vi "generate_RT_average.vi"(2 "Data In":T4, 7 "Variables Cluster":T2) -> (13 "Complete Data Out":T1, 15 "error out":errorcluster)   [LabVIEW 2023]
panel:
  out "C2 RT Avg Data":T3
  out "C1 RT Avg Data":T3
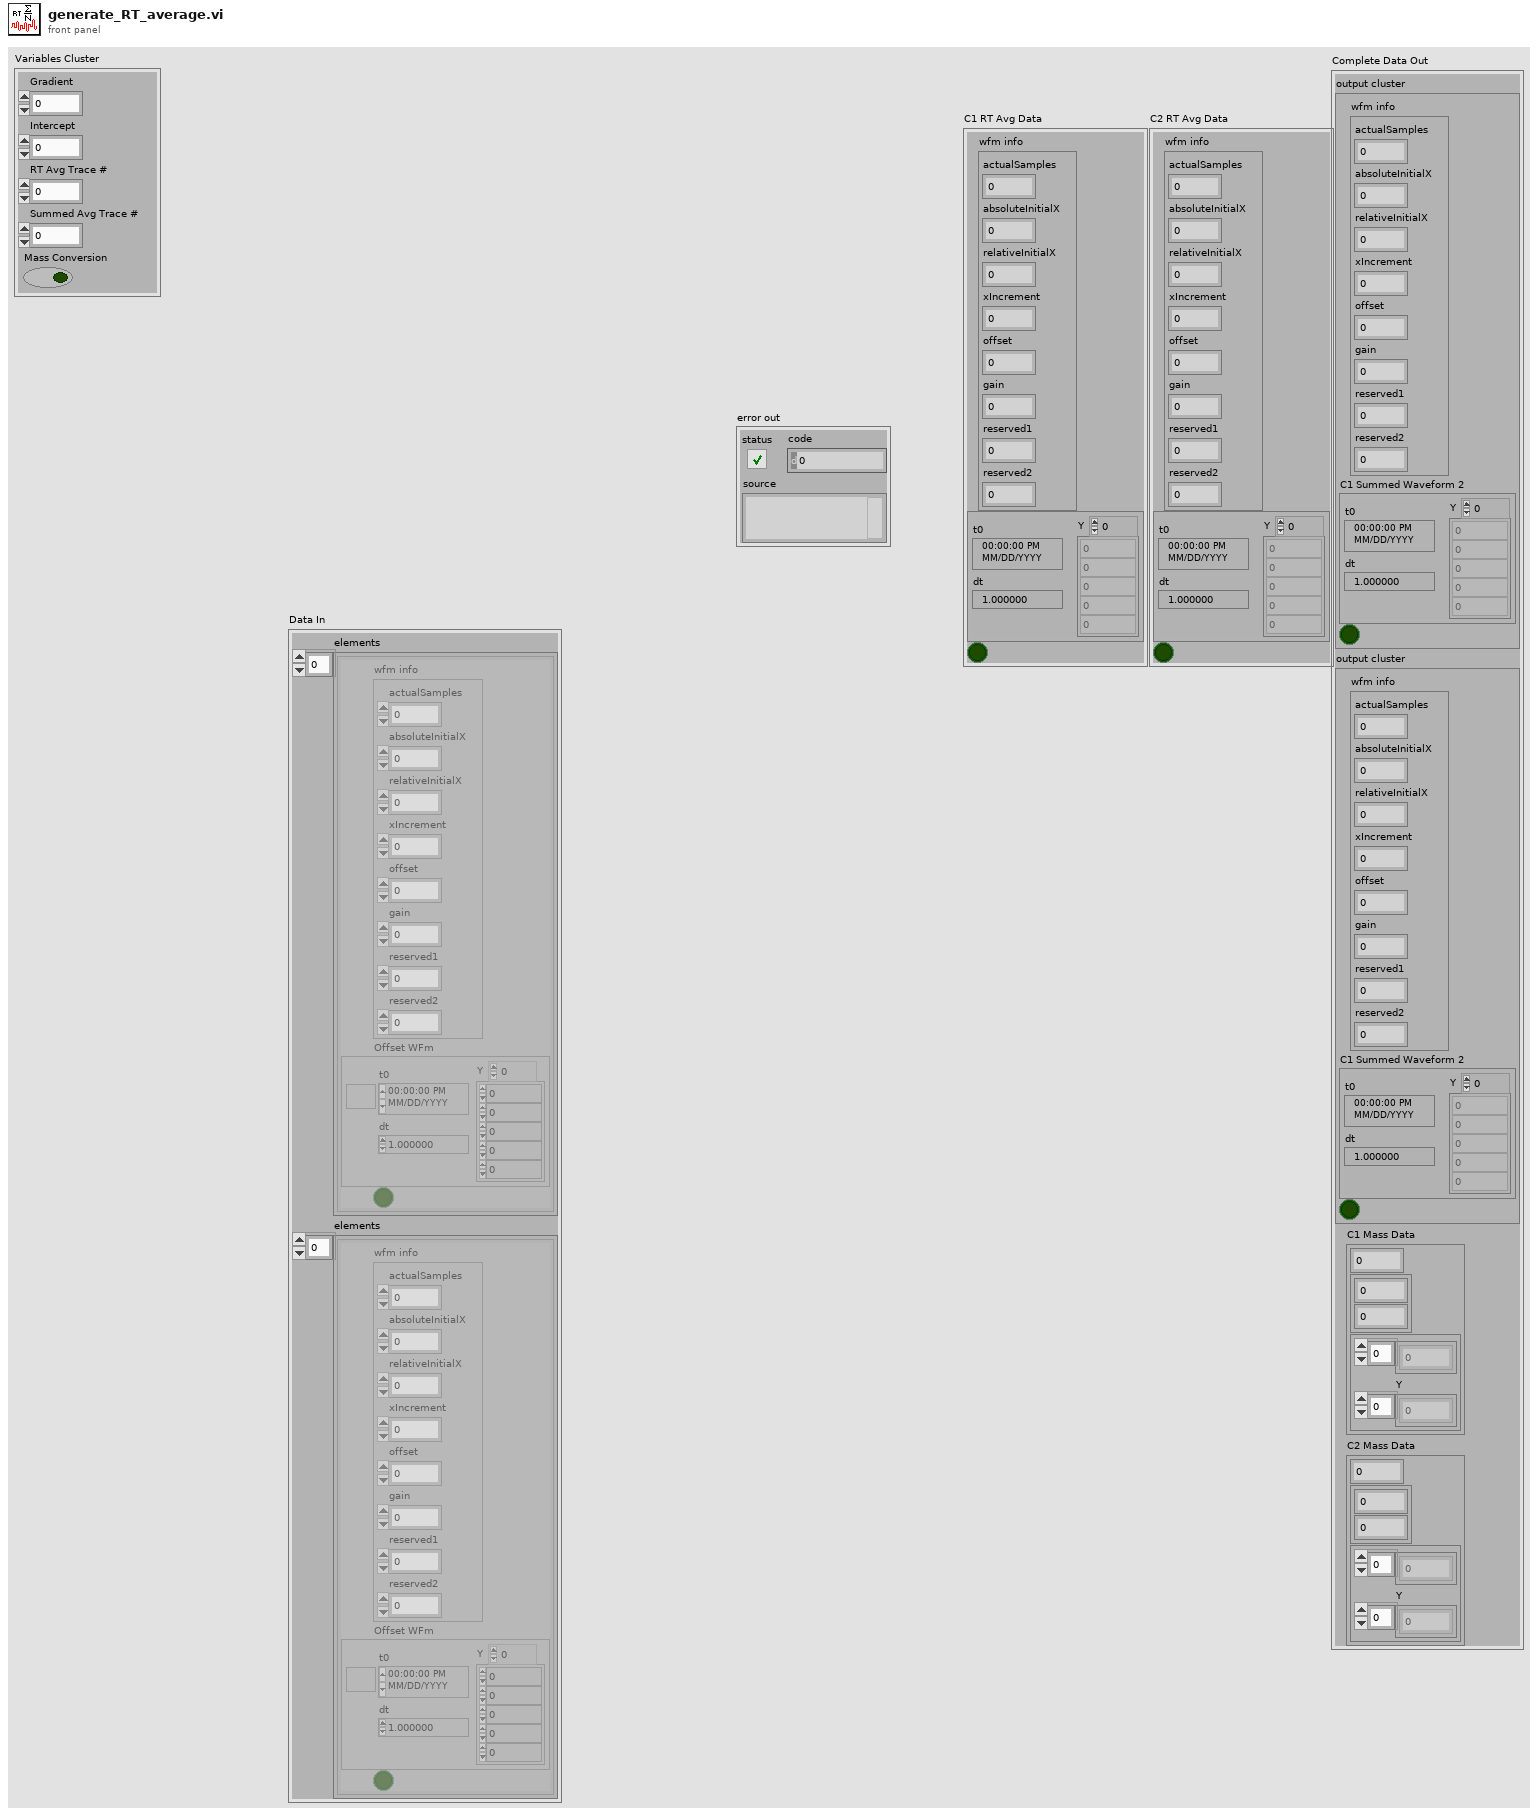
[diagram p1: front panel]
types:
  T1 = cluster{"output cluster":cluster{"wfm info":cluster{"actualSamples":i32, "absoluteInitialX":dbl, "relativeInitialX":dbl, "xIncrement":dbl, "offset":dbl, "gain":dbl, "reserved1":dbl, "reserved2":dbl}, "C1 Summed Waveform 2":waveform(dbl), bool}, "output cluster":cluster{"wfm info":cluster{"actualSamples":i32, "absoluteInitialX":dbl, "relativeInitialX":dbl, "xIncrement":dbl, "offset":dbl, "gain":dbl, "reserved1":dbl, "reserved2":dbl}, "C1 Summed Waveform 2":waveform(dbl), bool}, "C1 Mass Data":cluster{dbl, cluster{dbl, dbl}, cluster{dbl[], "Y":dbl[]}}, "C2 Mass Data":cluster{dbl, cluster{dbl, dbl}, cluster{dbl[], "Y":dbl[]}}}
  T2 = cluster{"Gradient":dbl, "Intercept":dbl, "RT Avg Trace #":i32, "Summed Avg Trace #":i32, "Mass Conversion":bool}
  T3 = cluster{"wfm info":cluster{"actualSamples":i32, "absoluteInitialX":dbl, "relativeInitialX":dbl, "xIncrement":dbl, "offset":dbl, "gain":dbl, "reserved1":dbl, "reserved2":dbl}, "Waveform":waveform(dbl), bool}
  T4 = cluster{"elements":cluster{"wfm info":cluster{"actualSamples":i32, "absoluteInitialX":dbl, "relativeInitialX":dbl, "xIncrement":dbl, "offset":dbl, "gain":dbl, "reserved1":dbl, "reserved2":dbl}, "Offset WFm":waveform(dbl), bool}[], "elements":cluster{"wfm info":cluster{"actualSamples":i32, "absoluteInitialX":dbl, "relativeInitialX":dbl, "xIncrement":dbl, "offset":dbl, "gain":dbl, "reserved1":dbl, "reserved2":dbl}, "Offset WFm":waveform(dbl), bool}[]}
  T5 = cluster{"wfm info":cluster{"actualSamples":i32, "absoluteInitialX":dbl, "relativeInitialX":dbl, "xIncrement":dbl, "offset":dbl, "gain":dbl, "reserved1":dbl, "reserved2":dbl}, "Offset WFm":waveform(dbl), bool}[]
  T6 = cluster{"actualSamples":i32, "absoluteInitialX":dbl, "relativeInitialX":dbl, "xIncrement":dbl, "offset":dbl, "gain":dbl, "reserved1":dbl, "reserved2":dbl}
  T7 = cluster{"wfm info":cluster{"actualSamples":i32, "absoluteInitialX":dbl, "relativeInitialX":dbl, "xIncrement":dbl, "offset":dbl, "gain":dbl, "reserved1":dbl, "reserved2":dbl}, waveform(dbl), bool}
  T8 = cluster{dbl, cluster{dbl, dbl}, cluster{dbl[], "Y":dbl[]}}
  T9 = cluster{cluster{"wfm info":cluster{"actualSamples":i32, "absoluteInitialX":dbl, "relativeInitialX":dbl, "xIncrement":dbl, "offset":dbl, "gain":dbl, "reserved1":dbl, "reserved2":dbl}, waveform(dbl), bool}, cluster{"wfm info":cluster{"actualSamples":i32, "absoluteInitialX":dbl, "relativeInitialX":dbl, "xIncrement":dbl, "offset":dbl, "gain":dbl, "reserved1":dbl, "reserved2":dbl}, waveform(dbl), bool}, "C1 Mass Data":cluster{dbl, cluster{dbl, dbl}, cluster{dbl[], "Y":dbl[]}}, "C2 Mass Data":cluster{dbl, cluster{dbl, dbl}, cluster{dbl[], "Y":dbl[]}}}
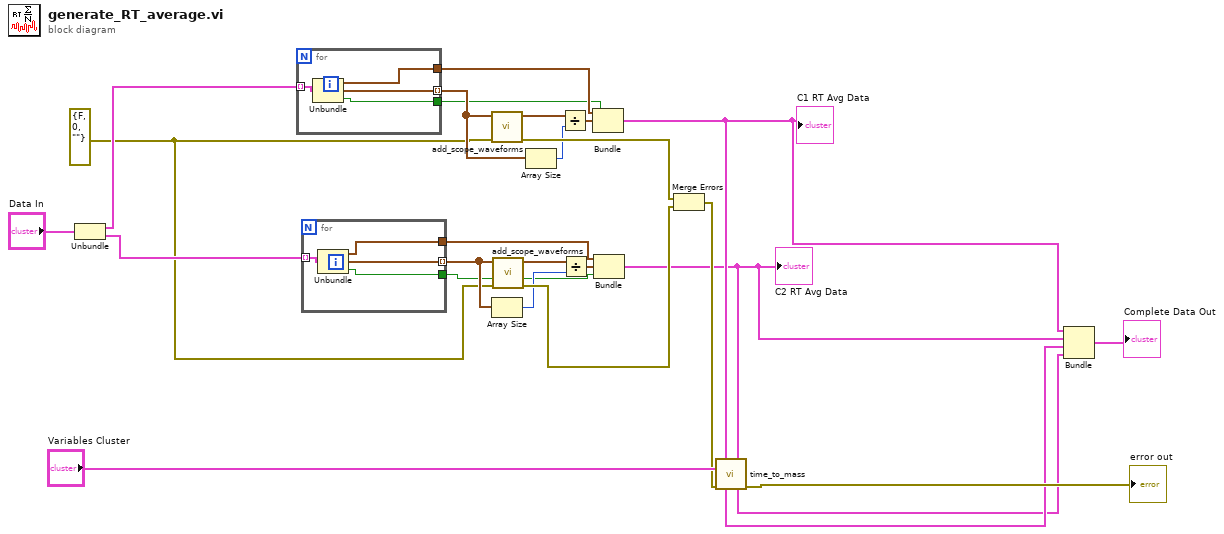
[diagram p0: block diagram]
diagram:
  w9 = errorcluster {"status"=FALSE, "code"=0, "source"=""} ("Error in (no error)")
  n1 = Unbundle("Data In") -> ("elements"=w26:T5, "elements"=w25:T5)
  n2 = for {
    tunnel: w26 -> [w30] mode=indexing
    tunnel: [w29] -> w20 mode=indexing
    tunnel: [w27] -> w17
    tunnel: [w28] -> w10
    n3 = Unbundle(w30) -> ("wfm info"=w27:T6, "Offset WFm"=w29:waveform(dbl), w28:bool)
  }
  n4 = for {
    tunnel: w25 -> [w34] mode=indexing
    tunnel: [w33] -> w15 mode=indexing
    tunnel: [w32] -> w12
    tunnel: [w31] -> w11
    n5 = Unbundle(w34) -> ("wfm info"=w32:T6, "Offset WFm"=w33:waveform(dbl), w31:bool)
  }
  n6 = call "add_scope_waveforms.vi"("Error in (no error)"=w9, "Waveform array"=w20) -> ("Error out"=w24:errorcluster, "Summed waveform"=w21:waveform(dbl))  [unwired: 8 in]
  n7 = Array Size(array=w15) -> (size(s)=w14:i32)
  n8 = call "add_scope_waveforms.vi"("Error in (no error)"=w9, "Waveform array"=w15) -> ("Error out"=w23:errorcluster, "Summed waveform"=w16:waveform(dbl))  [unwired: 8 in]
  n9 = Array Size(array=w20) -> (size(s)=w19:i32)
  n10 = Divide(x=w21, y=w19) -> (x/y=w18:waveform(dbl))
  n11 = Divide(x=w16, y=w14) -> (x/y=w13:waveform(dbl))
  n12 = Bundle("wfm info"=w17, w18, w10) -> (w5:T7)  [unwired: 1 in]
  "C1 RT Avg Data" <- w5
  n13 = Bundle("wfm info"=w12, w13, w11) -> (w4:T7)  [unwired: 1 in]
  "C2 RT Avg Data" <- w4
  n14 = Merge Errors(w24, w23) -> (w7:errorcluster)
  n15 = call "time_to_mass.vi"("C1 Data"=w5, "C2 Data"=w4, "Vairables Cluster"="Variables Cluster", "error in (no error)"=w7) -> ("C1 Mass Data"=w3:T8, "C2 Mass Data"=w2:T8, "error out"=→"error out":errorcluster)  [unwired: 9 in]
  n16 = Bundle(w5, w4, "C1 Mass Data"=w3, "C2 Mass Data"=w2) -> (→"Complete Data Out":T9)  [unwired: 1 in]
